vi "NMEA_ParseMessage-GPVTG.vi"(9 "Error In":errorcluster, 10 "$GPVTG-message_IN":string) -> (1 "Error Out":errorcluster, 2 "$GPVTG-message_OUT":T1={"True Course over Ground"=0.0, "Magnetic Course over Ground"=0.0, "Speed over Ground in knots"=0.0, "Speed over Ground in km/h"=1.0, "Mode"=""} {"Speed over Ground in km/h" format="%.02f [km/h]"; "Speed over Ground in knots" format="%.02f [kts]"; "Magnetic Course over Ground" format="%.02f [deg]"; "True Course over Ground" format="%.02f [deg]"})   [LabVIEW 2020, in "NMEA.lvlib"]
doc: "<B>GPVTG</B>\nTrack Made Good and Ground Speed"
uses:
  NMEA.lvlib
  NMEA_GPVTG-data.ctl
  NMEA_Mode.ctl
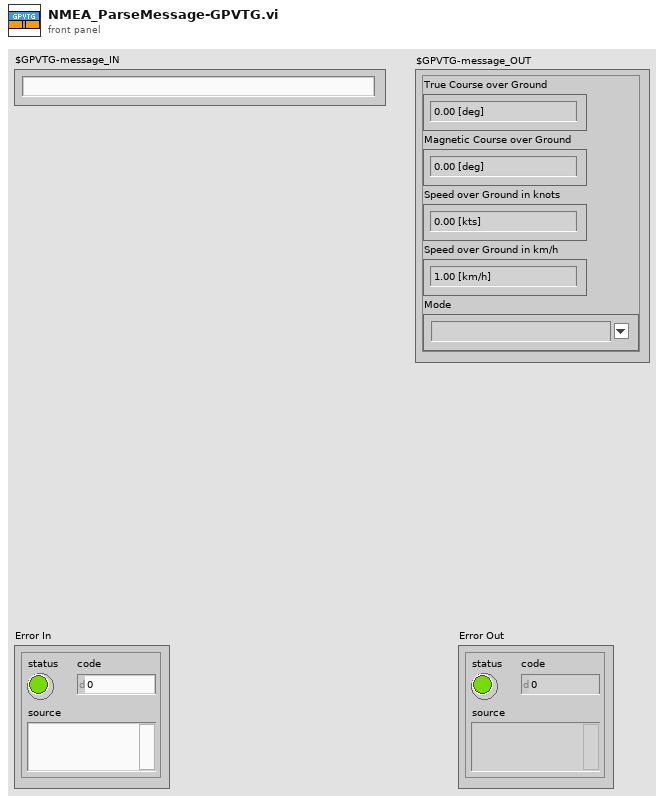
[diagram p1: front panel]
types:
  T1 = typedef "NMEA.lvlib/NMEA_GPVTG-data.ctl" = cluster{"True Course over Ground":dbl, "Magnetic Course over Ground":dbl, "Speed over Ground in knots":dbl, "Speed over Ground in km/h":dbl, "Mode":T2}
  T2 = typedef "NMEA.lvlib/NMEA_Mode.ctl" = string
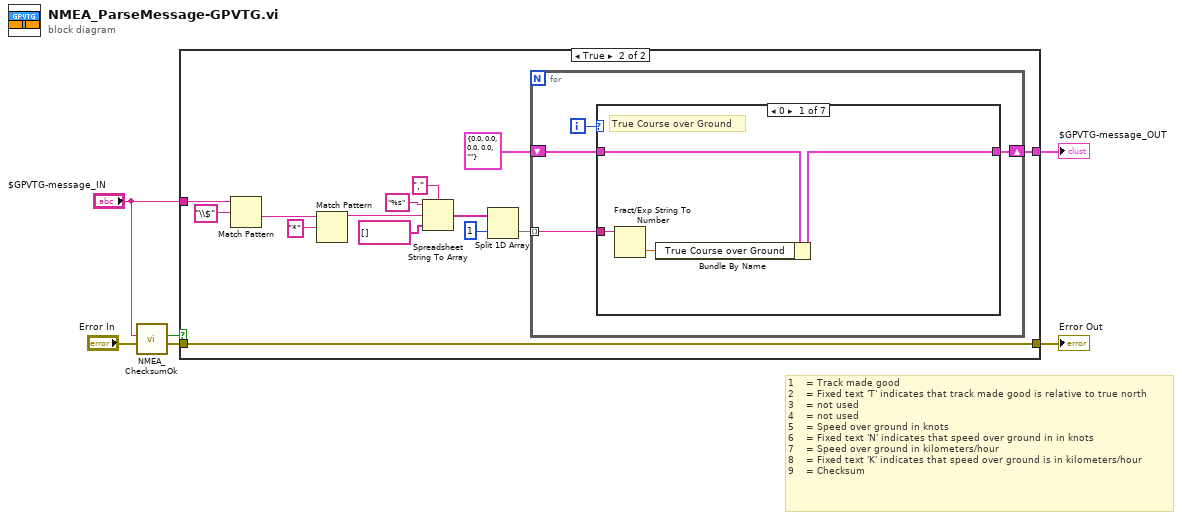
[diagram p0: block diagram]
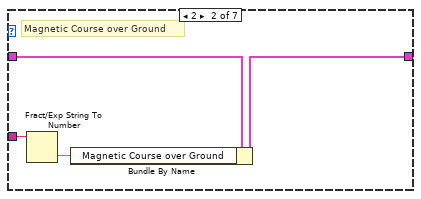
[diagram p3: hidden frame]
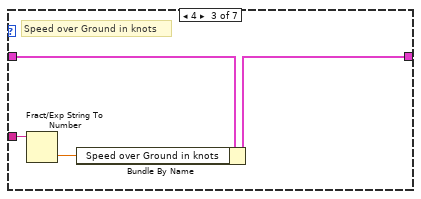
[diagram p4: hidden frame]
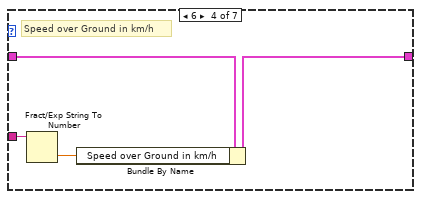
[diagram p5: hidden frame]
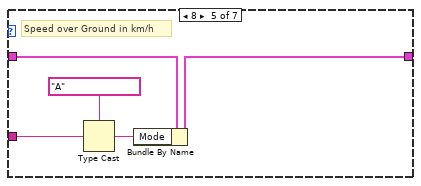
[diagram p6: hidden frame]
diagram:
  # "1    = Track made good\n2    = Fixed text 'T' indicates that track made good is relative to true north\n3    = not used\n4    = not used\n5    = Speed over ground in knots\n6    = Fixed text 'N' indicates that speed over ground in in knots\n7    = Speed over ground in kilometers/hour\n8    = Fixed text 'K' indicates that speed over ground is in kilometers/hour\n9    = Checksum"
  n1 = call "NMEA_ChecksumOk.vi"("Error In"="Error In", "Sentence"="$GPVTG-message_IN") -> ("Error Out"=w1:errorcluster, "CheckSumOk?"=w4:bool)  [unwired: 8 in]
  n2 = case shown="True" w4 {
    tunnel: [_ w16] -> w6
    tunnel: "$GPVTG-message_IN" -> [_ w14]
    tunnel: w1 -> [w7 w9]
    tunnel: [w7 w9] -> w3
    frame False {
    }
    frame True {
      n3 = Match Pattern(string=w14, regular expression="\\$") -> (after substring=w13:string)  [unwired: 1 in, 3 out]
      n4 = Match Pattern(string=w13, regular expression="*") -> (before substring=w20:string)  [unwired: 1 in, 3 out]
      n5 = Spreadsheet String To Array(delimiter (Tab)=",", format string="%s", spreadsheet string=w20, array type (2D Dbl)=string[] []) -> (array=w11:string[])
      n6 = Split 1D Array(array=w11, index=1) -> (second subarray=w12:string[])  [unwired: 1 out]
      n7 = for {
        tunnel: w12 -> [w22] mode=indexing
        shift-right: [w24] -> w16
        shift-left: T1 {"True Course over Ground"=0.0, "Magnetic Course over Ground"=0.0, "Speed over Ground in knots"=0.0, "Speed over Ground in km/h"=0.0, "Mode"=""} ("$GPVTG-message_OUT") -> [w25]
        i -> [w23]
        n8 = case shown="0" w23 {
          tunnel: w25 -> [w29 w33 w37 w41 w46 w47 w48]
          tunnel: [w28 w32 w36 w40 w45 w47 w48] -> w24
          tunnel: w22 -> [w27 w31 w35 w39 w43 _ _]
          frame 0 {
            # "True Course over Ground"
            n9 = Fract/Exp String To Number(string=w27) -> (number=w26:dbl)  [unwired: 3 in, 1 out]
            n10 = Bundle By Name(cluster=w29, "True Course over Ground"=w26) -> (w28:T1)
          }
          frame 2 {
            # "Magnetic Course over Ground"
            n11 = Fract/Exp String To Number(string=w31) -> (number=w30:dbl)  [unwired: 3 in, 1 out]
            n12 = Bundle By Name(cluster=w33, "Magnetic Course over Ground"=w30) -> (w32:T1)
          }
          frame 4 {
            # "Speed over Ground in knots"
            n13 = Fract/Exp String To Number(string=w35) -> (number=w34:dbl)  [unwired: 3 in, 1 out]
            n14 = Bundle By Name(cluster=w37, "Speed over Ground in knots"=w34) -> (w36:T1)
          }
          frame 6 {
            # "Speed over Ground in km/h"
            n15 = Fract/Exp String To Number(string=w39) -> (number=w38:dbl)  [unwired: 3 in, 1 out]
            n16 = Bundle By Name(cluster=w41, "Speed over Ground in km/h"=w38) -> (w40:T1)
          }
          frame 8 {
            # "Speed over Ground in km/h"
            n17 = Type Cast(type=T2 "A" ("Mode"), x=w43) -> (*(type *) &x=w42:T2)
            n18 = Bundle By Name(cluster=w46, "Mode"=w42) -> (w45:T1)
          }
          frame 1, 3, 5, 7 {
            # "[1] - True course over ground indicator (always 'T')\n[3] - Magnetic course over ground indicator (always 'M')\n[5] - Speed over ground in knots indicator (always 'N')\n[7] - Speed over ground in km/h indicator (always 'K')"
          }
          frame Default {
          }
        }
      }
    }
  }
  "$GPVTG-message_OUT" <- w6
  "Error Out" <- w3
